vi "Cannon Logic.vi"(1 "Cannon Info In":T2) -> (0 "Cannon Info Out?":T2)   [LabVIEW 2013]
uses:
  <vilib>/Rock Robotics/WPI/Solenoid/WPI_SolenoidValue.ctl
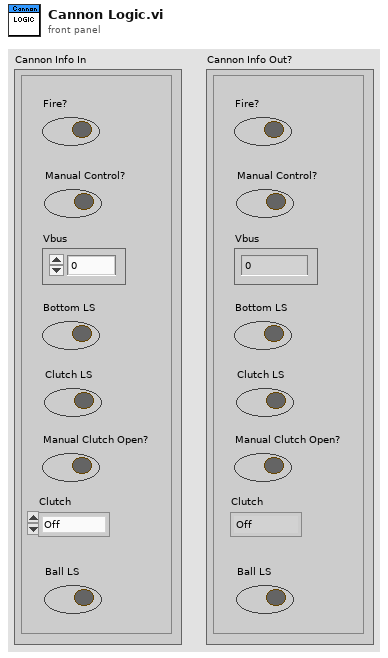
[diagram p1: front panel]
types:
  T1 = typedef "WPI_SolenoidValue.ctl" = enum16{"Off", "On", "Forward", "Reverse"}
  T2 = cluster{"Fire?":bool, "Manual Control?":bool, "Vbus":dbl, "Bottom LS":bool, "Clutch LS ":bool, "Manual Clutch Open?":bool, "Clutch":T1, "Ball LS":bool}
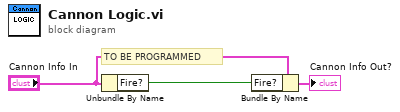
[diagram p0: block diagram]
diagram:
  # "TO BE PROGRAMMED"
  n1 = Unbundle By Name("Cannon Info In") -> ("Fire?"=w1:bool)
  n2 = Bundle By Name(cluster="Cannon Info In", "Fire?"=w1) -> (→"Cannon Info Out?":T2)
